vi "zero_crossing.vi"(9 "N":i32, 10 "freqs":dbl[](array[numeric]), 11 "derivative":dbl[](array[numeric])) -> (3 "zero_pos":dbl[](array[numeric]))   [LabVIEW 2018]
uses:
  <vilib>/Analysis/NI_AALPro.lvlib
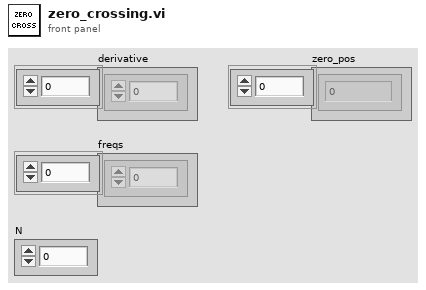
[diagram p1: front panel]
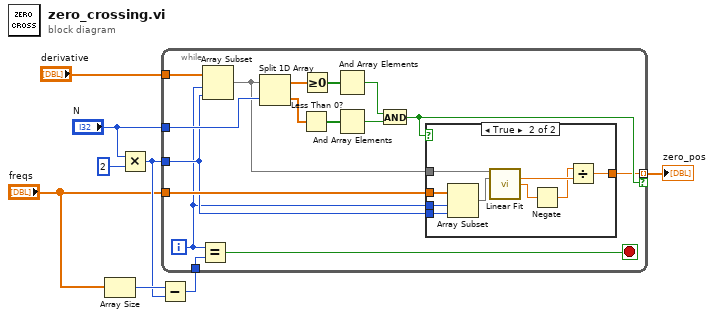
[diagram p0: block diagram]
diagram:
  n1 = Array Size(array="freqs") -> (size(s)=w5:i32)
  n2 = Multiply(x="N", y=2 ("x")) -> (x*y=w4:i32)
  n3 = Subtract(x=w5, y=w4) -> (x-y=w3:i32)
  n4 = while {
    tunnel: "derivative" -> [w24]
    tunnel: [w9] -> w1 mode=indexing if=w10
    tunnel: "freqs" -> [w14]
    tunnel: "N" -> [w23]
    tunnel: w4 -> [w13]
    tunnel: w3 -> [w22]
    i -> [w12]
    stop <- w21 stop-if-true
    n5 = Equal?(x=w12, y=w22) -> (x = y?=w21:bool)
    n6 = Array Subset(array=w24, index=w12, length=w13) -> (w11:dbl[])
    n7 = Split 1D Array(array=w11, index=w23) -> (first subarray=w20:dbl[], second subarray=w19:dbl[])
    n8 = Less Than 0?(x=w19) -> (x < 0?=w18:bool[])
    n9 = Greater Or Equal To 0?(x=w20) -> (x >= 0?=w17:bool[])
    n10 = And Array Elements(Boolean array=w17) -> (logical AND=w15:bool)
    n11 = And Array Elements(Boolean array=w18) -> (logical AND=w16:bool)
    n12 = And(x=w15, y=w16) -> (x .and. y?=w10:bool)
    n13 = case shown="True" w10 {
      tunnel: w14 -> [_ w33]
      tunnel: w13 -> [_ w32]
      tunnel: w12 -> [_ w31]
      tunnel: w11 -> [_ w29]
      tunnel: [_ w25] -> w9
      frame False {
      }
      frame True {
        n14 = Array Subset(array=w33, index=w31, length=w32) -> (w30:dbl[])
        n15 = call <vilib>:"Linear Fit.vi"("Y"=w29, "X"=w30) -> ("slope"=w27:dbl, "intercept"=w28:dbl)  [unwired: 9 in, 3 out]
        n16 = Negate(x=w28) -> (-x=w26:dbl)
        n17 = Divide(x=w26, y=w27) -> (x/y=w25:dbl)
      }
    }
  }
  "zero_pos" <- w1
